vi "lsl pull chunk buf.vi"(0 "in":cluster{}, 1 "data_buffer":string, 2 "lengths_buffer":u32, 3 "timestamp_buffer":dbl, 4 "data_buffer_elements":u32, 5 "timestamp_buffer_elements":u32, 6 "timeout":dbl, 7 "error in (no error)":errorcluster, 8 "ec":i32) -> (18 "ec out":i32, 20 "in out":cluster{}, 21 "data_buffer out":string, 22 "lengths_buffer out":u32, 23 "timestamp_buffer out":dbl, 24 "function return":u32, 27 "error out":errorcluster)   [LabVIEW 2018, in "liblsl-LabVIEW.lvlib"]
doc: "extern LIBLSL_C_API unsigned long lsl_pull_chunk_buf(lsl_inlet in, char **data_buffer, uint32_t *lengths_buffer, double *timestamp_buffer, unsigned long data_buffer_elements, unsigned long timestamp_buffer_elements, double timeout, int32_t *ec);"
uses:
  <userlib>/liblsl-LabVIEW/liblsl-LabVIEW.lvlib
  <userlib>/liblsl-LabVIEW/liblsl64.dll
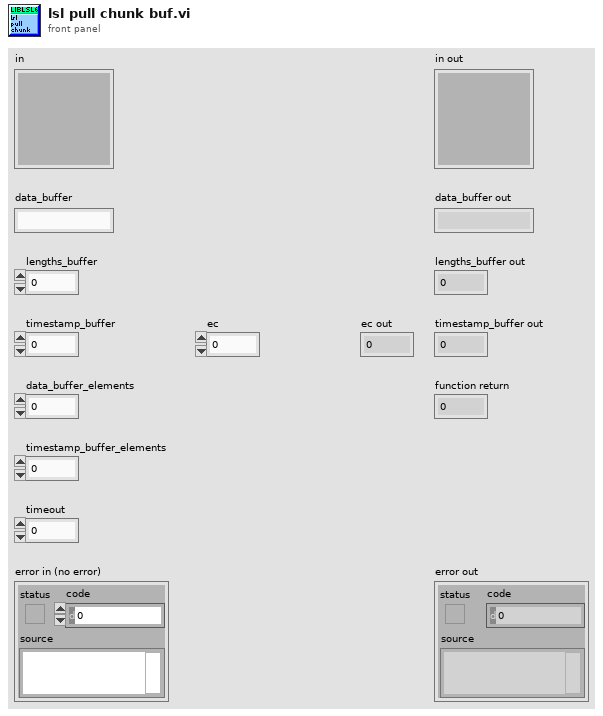
[diagram p1: front panel]
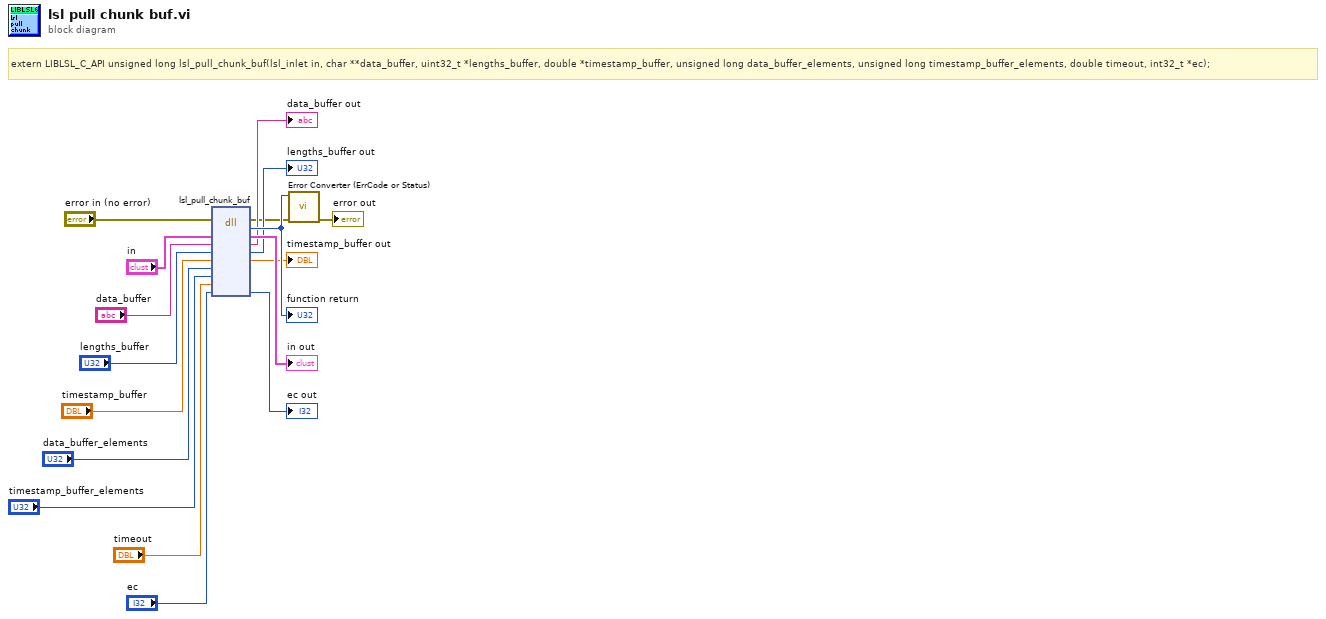
[diagram p0: block diagram]
diagram:
  # "extern LIBLSL_C_API unsigned long lsl_pull_chunk_buf(lsl_inlet in, char **data_buffer, uint32_t *lengths_buffer, double *timestamp_buffer, unsigned long data_buffer_elements, unsigned long timestamp_buffer_elements, double timeout, int32_t *ec);"
  n1 = dll-call lib="C:/Program Files/National Instruments/LabVIEW 2018/user.lib/liblsl-LabVIEW/liblsl64.*" fn="lsl_pull_chunk_buf"(error in="error in (no error)", "in"="in", "data_buffer"="data_buffer", "lengths_buffer"="lengths_buffer", "timestamp_buffer"="timestamp_buffer", "data_buffer_elements"="data_buffer_elements", "timestamp_buffer_elements"="timestamp_buffer_elements", "timeout"="timeout", "ec"="ec") -> (error out=w2:errorcluster, w17:u32, "in"=→"in out":cluster{}, "data_buffer"=→"data_buffer out":string, "lengths_buffer"=→"lengths_buffer out":u32, "timestamp_buffer"=→"timestamp_buffer out":dbl, "ec"=→"ec out":i32)  [unwired: 5 in, 1 out]
  "function return" <- w17
  n2 = call <userlib>:"Error Converter (ErrCode or Status).vi"("error in (no error)"=w2, "error code"=w17) -> ("error out"=→"error out":errorcluster)  [unwired: 9 in]
